vi "TEMI880 Example.vi"() -> ()   [LabVIEW 2017]
uses:
  <vilib>/Instr/_visa.llb/VISA Configure Serial Port (Instr).vi
panel:
  out "checksum":string
  out "value 2":u32
  out "value 3":string
  out "value 1":u32
  out "value 4":string
  out "OK":string
  out "command":string
  out "address 2":string
  out "STX":string
  out "bytes read":u32
  out "read string":string
  in  "delay before read (ms)":u32=500
  in  "include checksum":bool=TRUE
  in  "register number":u8
  in  "paragraph number":u8
  in  "address":u8
  in  "baud rate":u32=9600
  in  "VISA resource name":refnum<visa-resource-name>="COM1"
  in  "data bits":u16=8 min=5 max=8 step=1
  in  "parity":u16(ring) items=["None", "Odd", "Even", "Mark", "Space"]
  in  "stop bits":u16(ring)=10 items=["1.0"=10, "1.5"=15, "2.0"=20]
  in  "flow control":u16(ring) items=["None"=0, "XON/XOFF"=1, "RTS/CTS"=2, "DTR/DSR"=4]
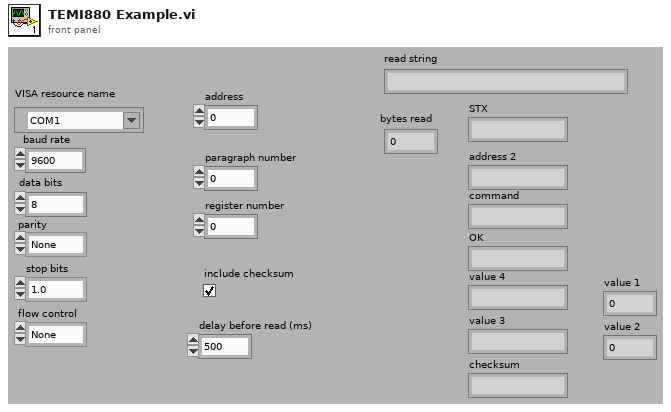
[diagram p1: front panel]
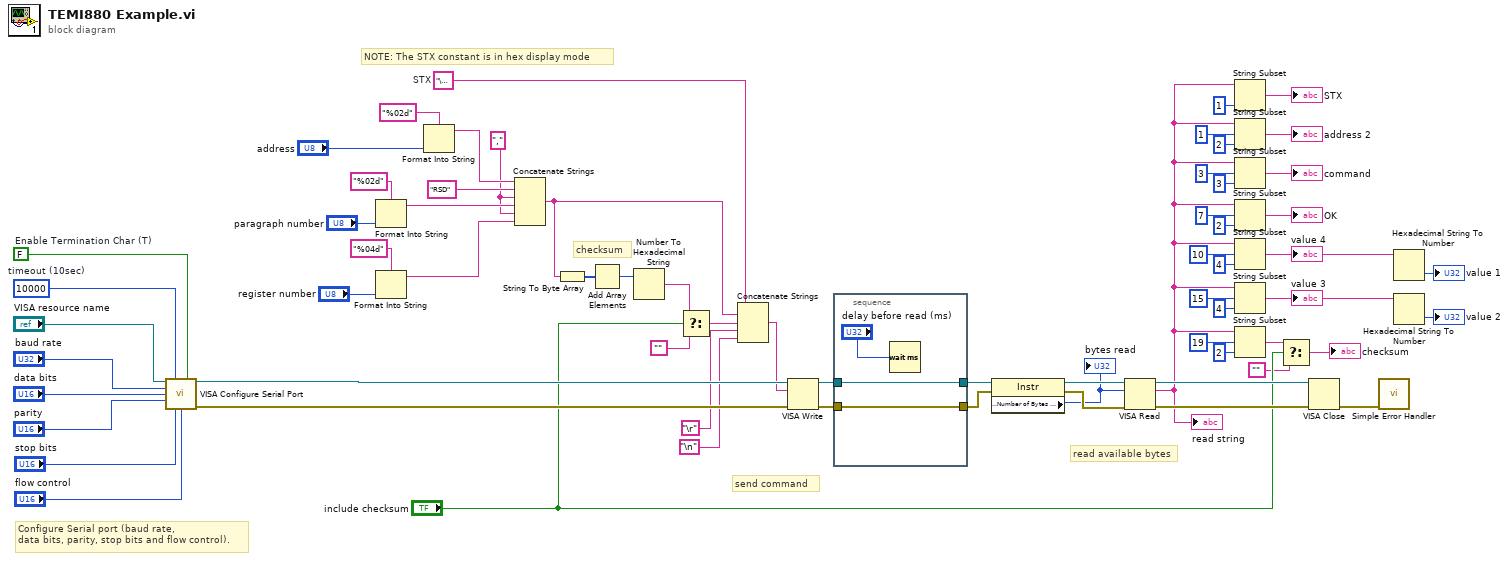
[diagram p0: block diagram]
diagram:
  w51 = "," ("format string")
  w43 = "\u0002"  # STX
  w64 = FALSE  # Enable Termination Char (T)
  w63 = u32 10000  # timeout (10sec)
  # "read available bytes"
  # "send command"
  # "checksum"
  # "NOTE: The STX constant is in hex display mode"
  # "Configure Serial port (baud rate,\ndata bits, parity, stop bits and flow control)."
  n1 = call-poly "VISA Configure Serial Port"("VISA resource name"="VISA resource name", "timeout (10sec)"=w63, "Enable Termination\nChar (T)"=w64, "baud rate (9600)"="baud rate", "data bits (8)"="data bits", "parity (0:none)"="parity", "stop bits (10: 1 bit)"="stop bits", "flow control (0:none)"="flow control") -> ("VISA resource name out"=w59:refnum<visa-resource-name>, "error out"=w58:errorcluster)  [unwired: 6 in]
  n2 = Format Into String(format string="%02d", "paragraph number") -> (resulting string=w52:string)  [unwired: 2 in, 1 out]
  n3 = Format Into String(format string="%04d", "register number") -> (resulting string=w47:string)  [unwired: 2 in, 1 out]
  n4 = Format Into String(format string="%02d", "address") -> (resulting string=w55:string)  [unwired: 2 in, 1 out]
  n5 = Concatenate Strings(w55, "RSD" ("format string"), w51, w52, w51, w47) -> (w27:string)
  n6 = String To Byte Array(string=w27) -> (unsigned byte array=w46:u8[])
  n7 = Add Array Elements(numeric array=w46) -> (sum=w44:u8)
  n8 = Number To Hexadecimal String(2:w44) -> (0:w42:string)  [unwired: 1 in]
  n9 = Select(t=w42, s="include checksum", f="") -> (s? t:f=w41:string)
  n10 = Concatenate Strings(w43, w27, w41, "\r", "\n") -> (w38:string)
  n11 = VISA Write(VISA resource name=w59, write buffer=w38, error in (no error)=w58) -> (VISA resource name out=w36:refnum<visa-resource-name>, error out=w37:errorcluster)  [unwired: 1 out]
  n12 = stacked-sequence {
    tunnel: w37 -> [w70]
    tunnel: [w70] -> w34
    tunnel: w36 -> [w69]
    tunnel: [w69] -> w35
    frame #0 {
      n13 = Wait (ms)(milliseconds to wait="delay before read (ms)") -> ()  [unwired: 1 out]
    }
  }
  n14 = property class="Instr"(reference=w35, error in=w34) -> (reference out=w33:refnum<visa-resource-name>, error out=w32:errorcluster, "Serial Settings:Number of Bytes at Serial Port"=w31:u32)
  "bytes read" <- w31
  n15 = VISA Read(VISA resource name=w33, byte count=w31, error in (no error)=w32) -> (VISA resource name out=w30:refnum<visa-resource-name>, read buffer=w5:string, error out=w29:errorcluster)  [unwired: 1 out]
  "read string" <- w5
  n16 = String Subset(string=w5, length (rest)=1 ("length (rest)")) -> (substring=→"STX":string)  [unwired: 1 in]
  n17 = String Subset(string=w5, offset (0)=1 ("length (rest)"), length (rest)=2 ("length (rest)")) -> (substring=→"address 2":string)
  n18 = String Subset(string=w5, offset (0)=3 ("length (rest)"), length (rest)=3 ("length (rest)")) -> (substring=→"command":string)
  n19 = String Subset(string=w5, offset (0)=7 ("length (rest)"), length (rest)=2 ("length (rest)")) -> (substring=→"OK":string)
  n20 = String Subset(string=w5, offset (0)=10 ("length (rest)"), length (rest)=4 ("length (rest)")) -> (substring=w13:string)
  "value 4" <- w13
  n21 = String Subset(string=w5, offset (0)=15 ("length (rest)"), length (rest)=4 ("length (rest)")) -> (substring=w10:string)
  "value 3" <- w10
  n22 = String Subset(string=w5, offset (0)=19 ("length (rest)"), length (rest)=2 ("length (rest)")) -> (substring=w3:string)
  n23 = Select(t=w3, s="include checksum", f="") -> (s? t:f=→"checksum":string)
  n24 = VISA Close(VISA resource name=w30, error in (no error)=w29) -> (error out=w28:errorcluster)
  n25 = call <vilib>:"Simple Error Handler.vi"("error in (no error)"=w28) -> ()  [unwired: 4 in, 5 out]
  n26 = Hexadecimal String To Number(string=w13) -> (number=→"value 1":u32)  [unwired: 2 in, 1 out]
  n27 = Hexadecimal String To Number(string=w10) -> (number=→"value 2":u32)  [unwired: 2 in, 1 out]
